vi "UdsLogCanRxMessage.vi"(0 "UdsHandleIn":T1, 2 "LogSuspend":bool, 5 "Id":u32 format="%08x", 7 "DataLength":u8, 9 "Data":u8[](array[numeric]) format="%02x", 11 "error in":errorcluster) -> (4 "UdsHandleOut":T1, 15 "error out":errorcluster)   [LabVIEW 2018, in "Konvolucio MUDS150628.lvlib"]
uses:
  Konvolucio MUDS150628.lvlib
  Types/UdsHandleType.ctl
  C:/Program Files/National Instruments/LabVIEW 2011/instr.lib/Konvolucio MCAN120803/Private/Konvolucio.MCAN120803.dll
  <instrlib>/Konvolucio MCAN120803/Types/MCanHandleType.ctl
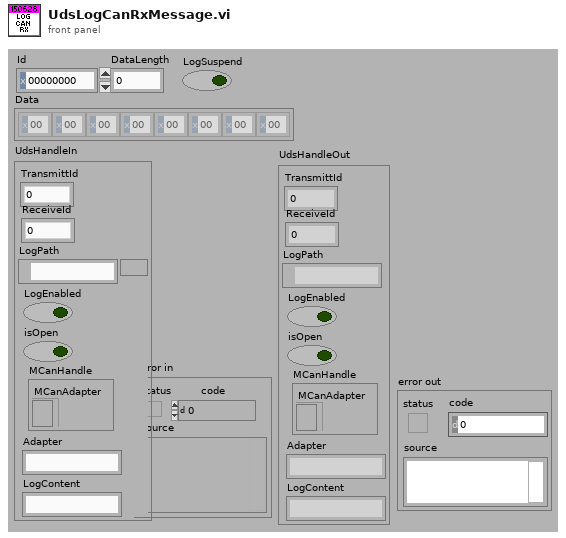
[diagram p1: front panel]
types:
  T1 = typedef "Konvolucio MUDS150628.lvlib/UdsHandleType.ctl" = cluster{"LogPath":path, "LogEnabled":bool, "isOpen":bool, "LogContent":string, "Adapter":string, "MCanHandle":T2, "TransmittId":u32, "ReceiveId":u32}
  T2 = typedef "Konvolucio MCAN120803.lvlib/MCanHandleType.ctl" = cluster{"MCanAdapter":refnum<k24>}
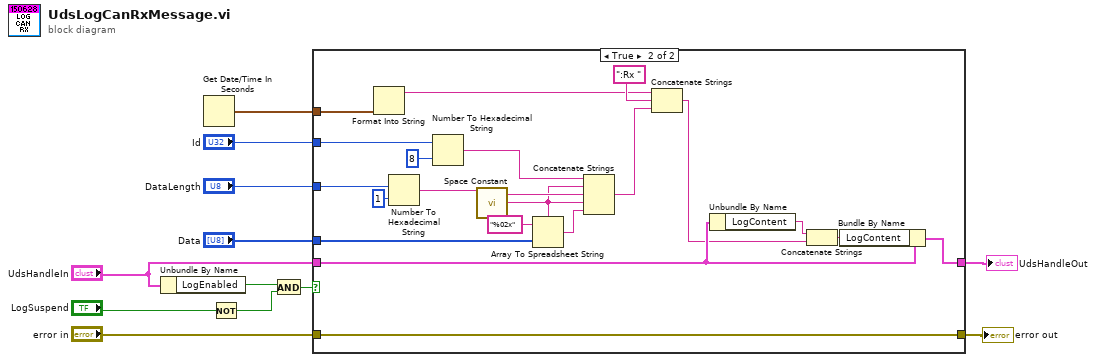
[diagram p0: block diagram]
diagram:
  n1 = Unbundle By Name("UdsHandleIn") -> ("LogEnabled"=w6:bool)
  n2 = Get Date/Time In Seconds() -> (seconds since 1Jan1904=w1:timestamp)
  n3 = Not(x="LogSuspend") -> (.not. x?=w4:bool)
  n4 = And(x=w6, y=w4) -> (x .and. y?=w3:bool)
  n5 = case shown="True" w3 {
    tunnel: "error in" -> [w14 w16]
    tunnel: [w14 w16] -> w11
    tunnel: [w13 w34] -> w9
    tunnel: "UdsHandleIn" -> [w13 w33]
    tunnel: "Data" -> [_ w23]
    tunnel: "DataLength" -> [_ w22]
    tunnel: "Id" -> [_ w20]
    tunnel: w1 -> [_ w18]
    frame False {
    }
    frame True {
      n6 = Format Into String(w18) -> (resulting string=w17:string)  [unwired: 3 in, 1 out]
      n7 = Number To Hexadecimal String(1:i16 1 ("width (-)"), 2:w22) -> (0:w29:string)
      n8 = Number To Hexadecimal String(1:i16 8 ("width (-)"), 2:w20) -> (0:w19:string)
      n9 = call <vilib>:"Space Constant.vi"() -> ("String"=w27:string)
      n10 = Array To Spreadsheet String(delimiter (Tab)=w27, array=w23, 3:"%02x" ("format string")) -> (spreadsheet string=w26:string)
      n11 = Concatenate Strings(w19, w27, w29, w27, w26) -> (w24:string)
      n12 = Concatenate Strings(w17, ":Rx " ("string"), w24) -> (w15:string)
      n13 = Unbundle By Name(w33) -> ("LogContent"=w31:string)
      n14 = Concatenate Strings(w31, w15) -> (w32:string)
      n15 = Bundle By Name(cluster=w33, "LogContent"=w32) -> (w34:T1)
    }
  }
  "error out" <- w11
  "UdsHandleOut" <- w9
